vi "RawDataAquisition.vi"(8 "error in":errorcluster, 9 "Sample Rate Fraction":i32, 10 "Sample Rate (samples / sec)":dbl, 11 "physical channels":tag) -> (0 "error out":errorcluster, 2 "Waveform Graph":dbl[][](graph))   [LabVIEW 2014]
uses:
  <vilib>/_DAQmxBase/Internals/DAQmxBase Create Channel (AI-Voltage-Basic).vi
  <vilib>/_DAQmxBase/Internals/DAQmxBase Timing (Sample Clock).vi
  <vilib>/_DAQmxBase/Internals/DAQmxBase Read (Analog 2D DBL NChan NSamp).vi
  <vilib>/Analysis/NI_AAL_SigProc.lvlib
panel:
  out "Locations":dbl[][](array[numeric])
  in  "peaks/valleys":enum32{"Peaks", "Valleys"}(ring)
  in  "width":i32(knob)=3 min=3 scale=3.0..16.0
  in  "Exit Button":bool
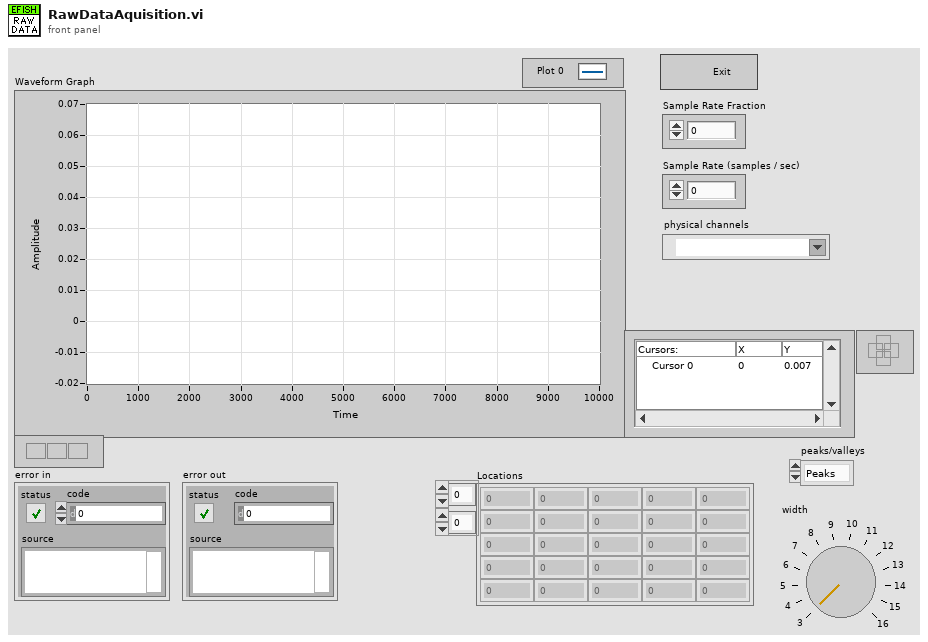
[diagram p1: front panel]
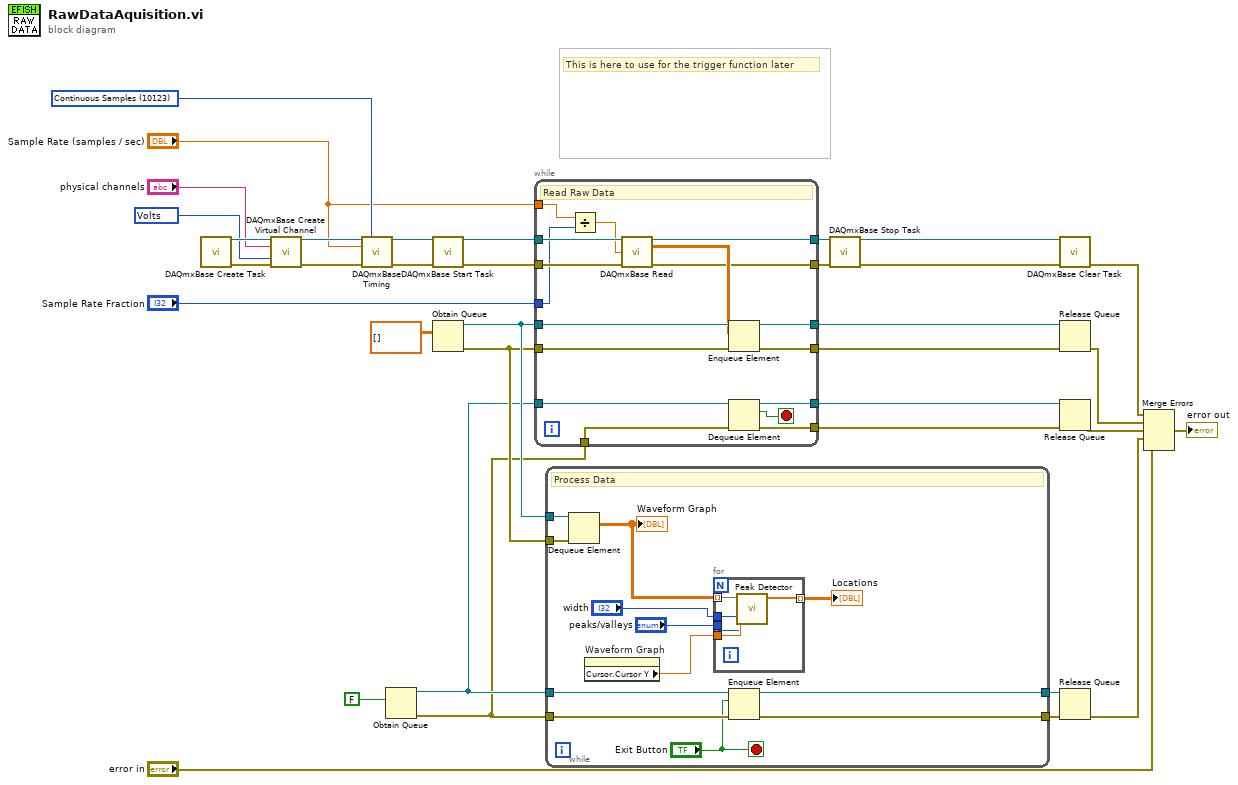
[diagram p0: block diagram]
diagram:
  w25 = 10123 items=["Finite Samples"=10178, "Continuous Samples"=10123, "Hardware Timed Single Point"=12522] ("sample mode")
  w28 = 10348 items=["Volts"=10348, "From Custom Scale"=10065] ("units")
  # "This is here to use for the trigger function later"
  n1 = call <vilib>:"DAQmxBase Create Task.vi"() -> ("task out"=w35:refnum<k21>, "error out"=w34:errorcluster)  [unwired: 14 in]
  n2 = call-poly <vilib>:"DAQmxBase Create Virtual Channel.vi"("task in"=w35, "physical channels"="physical channels", "units"=w28, "error in"=w34) -> ("task out"=w33:refnum<k21>, "error out"=w32:errorcluster)  [unwired: 10 in]
  n3 = call-poly <vilib>:"DAQmxBase Timing.vi"("task/channels in"=w33, "sample mode"=w25, "rate"="Sample Rate (samples / sec)", "error in"=w32) -> ("task out"=w31:refnum<k21>, "error out"=w30:errorcluster)  [unwired: 10 in]
  n4 = Obtain Queue(element data type=FALSE) -> (queue out=w19:refnum<queue>, error out=w18:errorcluster)  [unwired: 4 in, 1 out]
  n5 = call <vilib>:"DAQmxBase Start Task.vi"("task/channels in"=w31, "error in"=w30) -> ("task out"=w27:refnum<k21>, "error out"=w26:errorcluster)  [unwired: 12 in]
  n6 = Obtain Queue(element data type=dbl[][] []) -> (queue out=w22:refnum<queue>, error out=w21:errorcluster)  [unwired: 4 in, 1 out]
  n7 = while {
    tunnel: w22 -> [w52]
    tunnel: w21 -> [w51]
    tunnel: w27 -> [w50]
    tunnel: w26 -> [w49]
    tunnel: "Sample Rate Fraction" -> [w36]
    tunnel: w19 -> [w47]
    tunnel: w18 -> [w45]
    tunnel: "Sample Rate (samples / sec)" -> [w44]
    tunnel: [w42] -> w16
    tunnel: [w41] -> w15
    tunnel: [w40] -> w12
    tunnel: [w39] -> w11
    tunnel: [w38] -> w8
    tunnel: [w37] -> w7
    stop <- w46 stop-if-true
    # "Read Raw Data"
    n8 = Divide(x=w44, y=w36) -> (x/y=w43:dbl)
    n9 = call-poly <vilib>:"DAQmxBase Read.vi"("task/channels in"=w50, "number of samples per channel"=w43, "error in"=w49) -> ("task out"=w40:refnum<k21>, "data"=w48:dbl[][], "error out"=w39:errorcluster)  [unwired: 10 in]
    n10 = Enqueue Element(queue=w52, element=w48, error in (no error)=w51) -> (queue out=w38:refnum<queue>, error out=w37:errorcluster)  [unwired: 1 in, 1 out]
    n11 = Dequeue Element(queue=w47, error in (no error)=w45) -> (queue out=w42:refnum<queue>, element=w46:bool, error out=w41:errorcluster)  [unwired: 1 in, 1 out]
  }
  n12 = while {
    tunnel: w22 -> [w64]
    tunnel: w21 -> [w63]
    tunnel: w19 -> [w62]
    tunnel: w18 -> [w61]
    tunnel: [w59] -> w14
    tunnel: [w58] -> w13
    stop <- "Exit Button" stop-if-true
    # "Process Data"
    n13 = Dequeue Element(queue=w64, error in (no error)=w63) -> (element=w56:dbl[][])  [unwired: 1 in, 3 out]
    "Waveform Graph" <- w56
    n14 = property on="Waveform Graph" class="WFGraph (strict)"() -> ("Cursor.Cursor Y"=w57:dbl)  [unwired: 2 in, 2 out]
    n15 = for {
      tunnel: w57 -> [w69]
      tunnel: w56 -> [w68] mode=indexing
      tunnel: "width" -> [w67]
      tunnel: "peaks/valleys" -> [w66]
      tunnel: [w65] -> w53 mode=indexing
      n16 = call <vilib>:"Peak Detector.vi"("peaks/valleys"=w66, "width"=w67, "threshold"=w69, "X"=w68) -> ("Locations"=w65:dbl[])  [unwired: 3 in, 4 out]
    }
    "Locations" <- w53
    n17 = Enqueue Element(queue=w62, element="Exit Button", error in (no error)=w61) -> (queue out=w59:refnum<queue>, error out=w58:errorcluster)  [unwired: 1 in, 1 out]
  }
  n18 = call <vilib>:"DAQmxBase Stop Task.vi"("task/channels in"=w12, "error in"=w11) -> ("task out"=w10:refnum<k21>, "error out"=w9:errorcluster)  [unwired: 12 in]
  n19 = call <vilib>:"DAQmxBase Clear Task.vi"("task in"=w10, "error in"=w9) -> ("error out"=w6:errorcluster)  [unwired: 13 in]
  n20 = Release Queue(queue=w8, error in (no error)=w7) -> (error out=w5:errorcluster)  [unwired: 1 in, 2 out]
  n21 = Release Queue(queue=w16, error in (no error)=w15) -> (error out=w4:errorcluster)  [unwired: 1 in, 2 out]
  n22 = Release Queue(queue=w14, error in (no error)=w13) -> (error out=w3:errorcluster)  [unwired: 1 in, 2 out]
  n23 = Merge Errors(w6, w5, w4, w3, "error in") -> (→"error out":errorcluster)
